vi "ComputeShift.vi"(0 "X1":dbl format="%#_11g", 1 "Y1":dbl format="%#_11g", 2 "X2":dbl format="%#_10g", 3 "Y2":dbl format="%#_11g", 4 "Path":path) -> (7 "XShift":dbl format="%#_8g", 8 "YShift":dbl format="%#_8g", 9 "Length":dbl format="%#_9g")   [LabVIEW 2018]
uses:
  <vilib>/Utility/file.llb/Read Delimited Spreadsheet (DBL).vi
panel:
  out "Ux":dbl
  out "Uy":dbl
  out "X_cp":dbl format="%#_8g"
  out "Y_cp":dbl format="%#_8g"
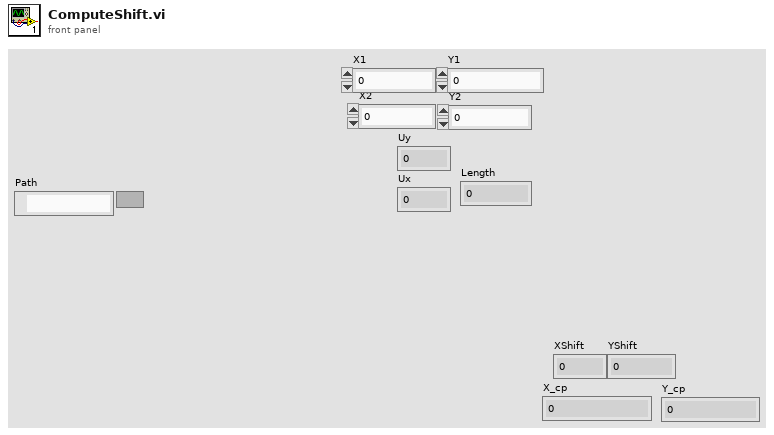
[diagram p1: front panel]
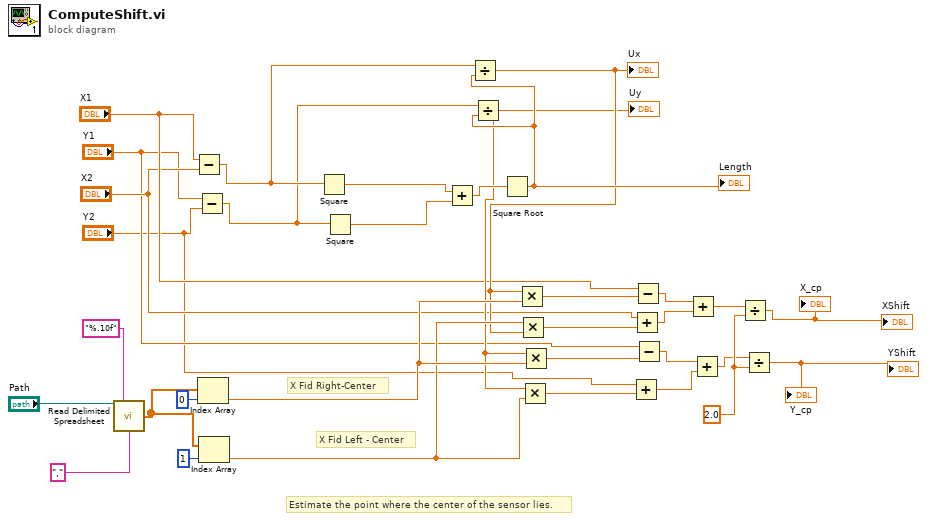
[diagram p0: block diagram]
diagram:
  w25 = 2.0 ("y")
  # "Estimate the point where the center of the sensor lies."
  # "X Fid Left - Center"
  # "X Fid Right-Center"
  n1 = call-poly <vilib>:"Read Delimited Spreadsheet.vi"("file path (dialog if empty)"="Path", "format (%.3f)"="%.10f", "delimiter (\\t)"="," ("delimiter (\\t)")) -> ("first row"=w17:dbl[])  [unwired: 7 in, 5 out]
  n2 = Subtract(x="X1", y="X2") -> (x-y=w9:dbl)
  n3 = Subtract(x="Y1", y="Y2") -> (x-y=w8:dbl)
  n4 = Index Array(array=w17, index=0) -> (element=w16:dbl)
  n5 = Index Array(array=w17, index=1) -> (element=w15:dbl)
  n6 = Square(x=w9) -> (x^2=w11:dbl)
  n7 = Square(x=w8) -> (x^2=w10:dbl)
  n8 = Add(x=w11, y=w10) -> (x+y=w12:dbl)
  n9 = Square Root(x=w12) -> (sqrt(x)=w7:dbl)
  "Length" <- w7
  n10 = Divide(x=w9, y=w7) -> (x/y=w6:dbl)
  "Ux" <- w6
  n11 = Divide(x=w8, y=w7) -> (x/y=w5:dbl)
  "Uy" <- w5
  n12 = Multiply(x=w6, y=w16) -> (x*y=w33:dbl)
  n13 = Multiply(x=w15, y=w6) -> (x*y=w32:dbl)
  n14 = Multiply(x=w5, y=w15) -> (x*y=w30:dbl)
  n15 = Multiply(x=w5, y=w16) -> (x*y=w31:dbl)
  n16 = Add(x="Y2", y=w30) -> (x+y=w26:dbl)
  n17 = Add(x="X2", y=w32) -> (x+y=w28:dbl)
  n18 = Subtract(x="X1", y=w33) -> (x-y=w29:dbl)
  n19 = Subtract(x="Y1", y=w31) -> (x-y=w27:dbl)
  n20 = Add(x=w29, y=w28) -> (x+y=w23:dbl)
  n21 = Add(x=w27, y=w26) -> (x+y=w24:dbl)
  n22 = Divide(x=w23, y=w25) -> (x/y=→"XShift" →"X_cp":dbl)
  n23 = Divide(x=w24, y=w25) -> (x/y=→"YShift" →"Y_cp":dbl)
